vi "CallbackHelp_MatrixMinus.vi"(9 "B":T1, 10 "A":T1, 11 "Variant":variant) -> (0 "Error":bool, 3 "Output":T1)   [LabVIEW 2019, in "Trajectory_Library.lvlib"]
doc: "matrix callback function that performs\n\n A - B\n\nInputs:\n - ExtraData -- Variant containing extra data -- not used\n - A -- A matrix\n - B -- B matrix\n\nOutputs:\n - Output -- Resulting matrix\n - Error -- If TRUE, an error occured."
uses:
  Trajectory_Library.lvlib
  <vilib>/Analysis/Matrix/Datatypes/RealMatrix.ctl
  <vilib>/Analysis/Matrix/Numeric/Subtract/Subtract - RM,RM.vi
  <vilib>/Analysis/Matrix/NI_Matrix.lvlib
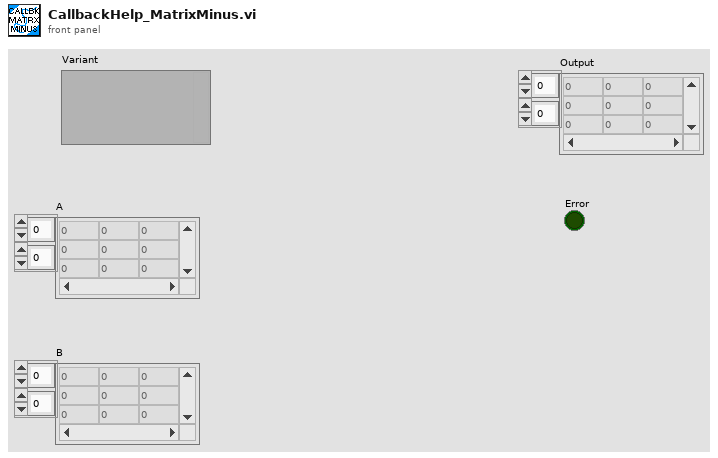
[diagram p1: front panel]
types:
  T1 = typedef "NI_Matrix.lvlib/RealMatrix.ctl" = dbl[][]
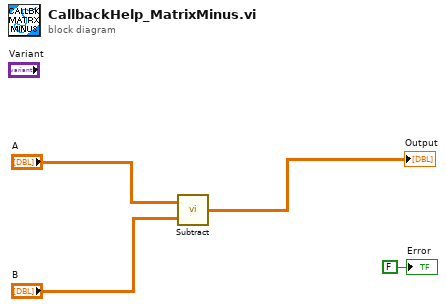
[diagram p0: block diagram]
diagram:
  n1 = call-poly <vilib>:"Subtract.vi"("Real Matrix B"="B", "Real Matrix A"="A") -> ("A - B"=→"Output":T1)
  "Error" <- FALSE ("Error")
